vi "error_status.vi"() -> ()   [LabVIEW 2013]
panel:
  out "status":string
  out "status":bool
  in  "error in (no error)":errorcluster
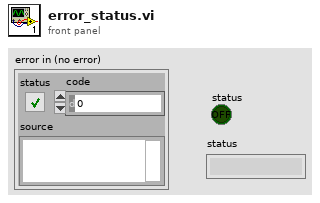
[diagram p1: front panel]
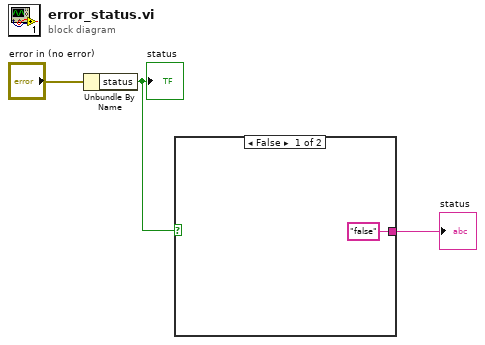
[diagram p0: block diagram]
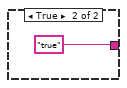
[diagram p2: hidden frame]
diagram:
  n1 = Unbundle By Name("error in (no error)") -> ("status"=w2:bool)
  "status" <- w2
  n2 = case shown="False" w2 {
    tunnel: ["false" "true"] -> w1
    frame False {
    }
    frame True {
    }
  }
  "status" <- w1
